vi "Test Namer With Folder Default Behavior.vi"(11 "Test Case In":refnum<class "Namer Tests.lvclass">) -> (0 "error out":errorcluster, 3 "Test Case Out":refnum<class "Namer Tests.lvclass">)   [LabVIEW 2020, in "Namer Tests.lvclass"]
uses:
  Namer Tests.lvclass
  C:/Program Files/National Instruments/LabVIEW 2026/vi.lib/Astemes/LUnit/Test Case.lvclass
  Source/Approval Tests/Namer with Folder/Namer with Folder.lvclass
  Source/Approval Tests/Naming Data/Naming Data.lvclass
  Source/Approval Tests/Naming Data/Naming Data.lvclass/Naming Data.ctl
  <vilib>/Astemes/LUnit/Test Case.lvclass/Test Case.ctl
  4993e8ee-a06a-463a-9684-69129f64d5ce.vi
  cbc5bbb8-e1dd-4019-9d94-c2b48c5ee7af.vi
  Source/Approval Tests/Naming Data/Write Test VI Name.vi
  <vilib>/Astemes/LUnit/Core/LUnit Test Case/Private/Append Pass Result.vi
  <vilib>/Astemes/LUnit/Core/LUnit Test Case/Private/Append Fail Result.vi
  4993e8ee-a06a-463a-9684-69129f64d5ce.vi/9c5d11cd-9439-4240-a1ee-d9baace9c924.vi
  cbc5bbb8-e1dd-4019-9d94-c2b48c5ee7af.vi/9c5d11cd-9439-4240-a1ee-d9baace9c924.vi
  <vilib>/Astemes/LUnit/Core/LUnit Test Case/Private/Run In UI.vi
  <vilib>/Utility/error.llb/Clear Errors.vi
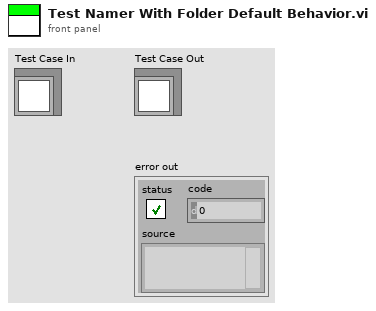
[diagram p1: front panel]
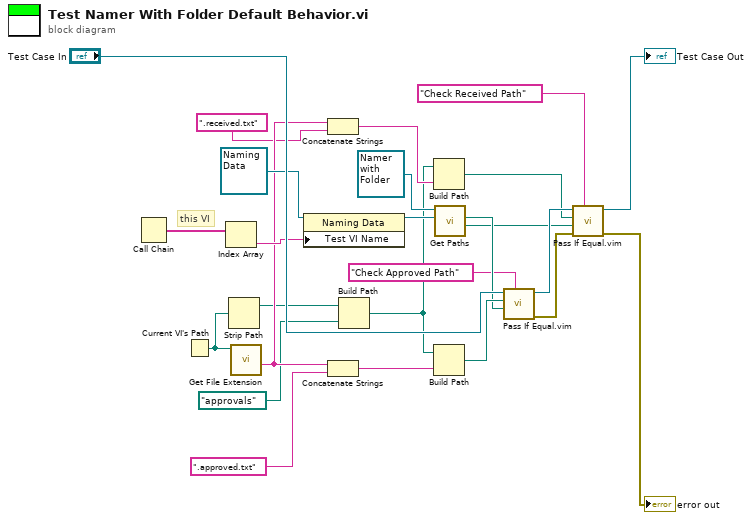
[diagram p0: block diagram]
diagram:
  # "this VI"
  n1 = Call Chain() -> (call chain=w20:string[])
  n2 = Current VI's Path() -> (path=w17:path)
  n3 = Index Array(array=w20) -> (element=w19:string)  [unwired: 1 in]
  n4 = Strip Path(path=w17) -> (stripped path=w10:path)  [unwired: 1 out]
  n5 = call <vilib>:"Get File Extension.vi"("file"=w17) -> ("filename without extension"=w16:string)  [unwired: 6 in, 4 out]
  n6 = property on="Property Node" class="Naming Data"(reference=refnum<class "Naming Data.lvclass"> refnum ("Naming Data"), "Test VI Name"=w19) -> (reference out=w18:refnum<class "Naming Data.lvclass">)  [unwired: 1 in, 1 out]
  n7 = Concatenate Strings(w16, ".received.txt" ("string")) -> (w13:string)
  n8 = Concatenate Strings(w16, ".approved.txt" ("string")) -> (w12:string)
  n9 = Build Path(base path=w10, name or relative path=path "approvals") -> (appended path=w11:path)
  n10 = Build Path(base path=w11, name or relative path=w13) -> (appended path=w4:path)
  n11 = Build Path(base path=w11, name or relative path=w12) -> (appended path=w8:path)
  n12 = call-dynamic "Get Paths.vi"("Naming Data"=w18, "Namer with Folder in"=refnum<class "Namer with Folder.lvclass"> refnum ("Approval Tests:Namer with SubFolder.lvclass")) -> ("Received Path"=w3:path, "Approved Path"=w7:path)  [unwired: 6 in, 2 out]
  n13 = call "Pass If Equal.vim"("Description"="Check Approved Path" ("Label (VI Title)"), "Actual"=w7, "Expected"=w8, "LUnit Test Case In"="Test Case In") -> ("error out"=w24:errorcluster, "LUnit Test Case Out"=w6:refnum<class "Namer Tests.lvclass">)  [unwired: 6 in]
  n14 = call "Pass If Equal.vim"("Description"="Check Received Path" ("Label (VI Title)"), "error in (no error)"=w24, "Actual"=w3, "Expected"=w4, "LUnit Test Case In"=w6) -> ("error out"=→"error out":errorcluster, "LUnit Test Case Out"=→"Test Case Out":refnum<class "Namer Tests.lvclass">)  [unwired: 5 in]
